vi "GetKeyboardInfo-SubVI.vi"(0 "Key Selections":T1, 1 "Key\nValue":u16) -> (2 "Key values":cluster{i32, i32, i32, i32, i32, i32, i32}, 3 "number":u32, 4 "Max Velocity Value":i32)   [LabVIEW 2014]
panel:
  out "X Decreasing (#)":i32
  out "Y Decreasing (#)":i32
  out "X Increasing (#)":i32
  out "Y Increasing (#)":i32
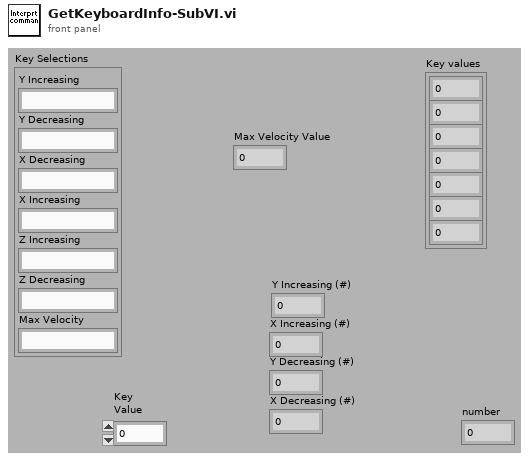
[diagram p1: front panel]
types:
  T1 = cluster{"Y Increasing":string, "Y Decreasing":string, "X Decreasing":string, "X Increasing":string, "Z Increasing":string, "Z Decreasing":string, "Max Velocity":string}
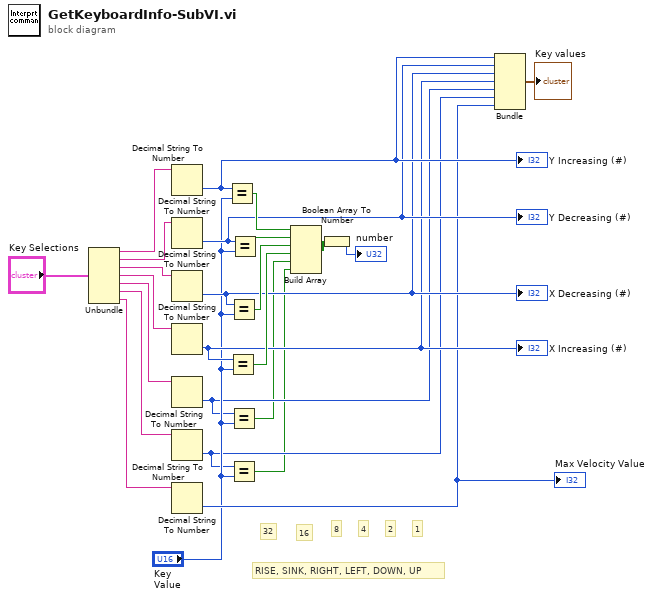
[diagram p0: block diagram]
diagram:
  # "32"
  # "16"
  # "8"
  # "4"
  # "2"
  # "1"
  # "RISE, SINK, RIGHT, LEFT, DOWN, UP"
  n1 = Unbundle("Key Selections") -> ("Y Increasing"=w15:string, "Y Decreasing"=w14:string, "X Decreasing"=w13:string, "X Increasing"=w12:string, "Z Increasing"=w8:string, "Z Decreasing"=w7:string, "Max Velocity"=w9:string)
  n2 = Decimal String To Number(string=w15) -> (number=w19:i32)  [unwired: 3 out]
  "Y Increasing (#)" <- w19
  n3 = Decimal String To Number(string=w14) -> (number=w18:i32)  [unwired: 3 out]
  "Y Decreasing (#)" <- w18
  n4 = Decimal String To Number(string=w13) -> (number=w17:i32)  [unwired: 3 out]
  "X Decreasing (#)" <- w17
  n5 = Decimal String To Number(string=w12) -> (number=w16:i32)  [unwired: 3 out]
  "X Increasing (#)" <- w16
  n6 = Decimal String To Number(string=w8) -> (number=w3:i32)  [unwired: 3 out]
  n7 = Decimal String To Number(string=w7) -> (number=w4:i32)  [unwired: 3 out]
  n8 = Decimal String To Number(string=w9) -> (number=w10:i32)  [unwired: 3 out]
  "Max Velocity Value" <- w10
  n9 = Equal?(x=w19, y="Key\nValue") -> (x = y?=w25:bool)
  n10 = Equal?(x=w16, y="Key\nValue") -> (x = y?=w22:bool)
  n11 = Equal?(x=w17, y="Key\nValue") -> (x = y?=w23:bool)
  n12 = Equal?(x=w3, y="Key\nValue") -> (x = y?=w2:bool)
  n13 = Equal?(x=w4, y="Key\nValue") -> (x = y?=w1:bool)
  n14 = Equal?(x=w18, y="Key\nValue") -> (x = y?=w24:bool)
  n15 = Build Array(w25, w24, w23, w22, w2, w1) -> (w21:bool[])
  n16 = Boolean Array To Number(Boolean array=w21) -> (number=→"number":u32)
  n17 = Bundle(w19, w18, w17, w16, w3, w4, w10) -> (→"Key values":cluster{i32, i32, i32, i32, i32, i32, i32})  [unwired: 1 out]
